vi "GPIB with VISA functions2.vi"() -> ()   [LabVIEW 2015]
doc: "本范例需要在系统中安装NI-488.2和NI-VISA。本范例演示了如何通过对返回数据使用VISA读取、写入和格式函数，与GPIB仪器进行通信。本范例可用于NI Instrument Simulator或其他类似仪器。"
panel:
  in  "波形":enum16{"SIN", "SQU", "RAND"}(ring)
  out "波形图":dbl[](graph)
  out "原始数据":string
  in  "VISA GPIB资源":refnum<visa-resource-name>="GPIB0::2::INSTR"
  # "概述：演示使用VISA函数与GPIB仪器进行通信的方法。\n要求：NI-488.2和NI-VISA驱动程序\n操作步骤：\n1. 请先在Measurement & Automation Explorer正确配置VISA GPIB资源控件中指定的资源。\n2. 运行VI。\n3.如仪器识别了\"SOUR:FUNC\"和\"SENS:DATA?\"命令，则应返回指定的波形数据。"
  # "Windows/Linux用户可使用“仪器驱动程序查找器”（帮助>查找仪器驱动）为仪器查找相应的驱动程序。"
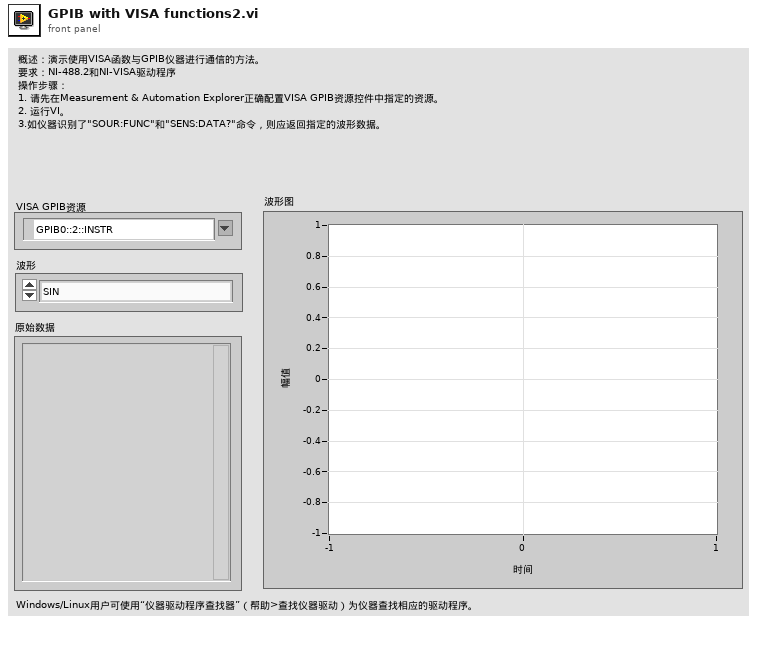
[diagram p1: front panel]
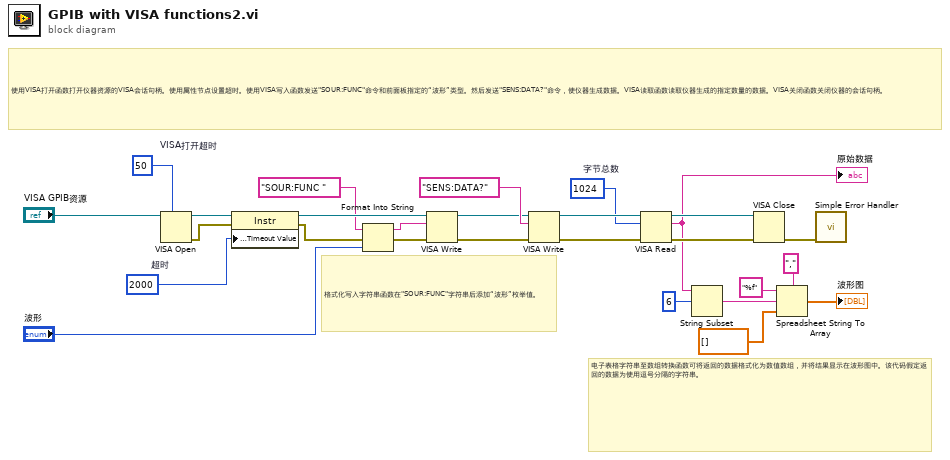
[diagram p0: block diagram]
diagram:
  w17 = u32 1024  # 字节总数
  w22 = u32 2000  # 超时
  w23 = u32 50  # VISA打开超时
  # "电子表格字符串至数组转换函数可将返回的数据格式化为数值数组，并将结果显示在波形图中。该代码假定返回的数据为使用逗号分隔的字符串。"
  # "格式化写入字符串函数在\"SOUR:FUNC\"字符串后添加“波形”枚举值。"
  # "使用VISA打开函数打开仪器资源的VISA会话句柄。使用属性节点设置超时。使用VISA写入函数发送\"SOUR:FUNC\"命令和前面板指定的“波形”类型。然后发送\"SENS:DATA?\"命令，使仪器生成数据。VISA读取函数读取仪器生成的指定数量的数据。VISA关闭函数关闭仪器的会话句柄。"
  n1 = VISA Open(timeout (0)=w23, VISA resource name="VISA GPIB资源") -> (VISA resource name=w21:refnum<visa-resource-name>, error out=w20:errorcluster)  [unwired: 3 in]
  n2 = property class="Instr"(reference=w21, error in=w20, "General Settings:Timeout Value"=w22) -> (reference out=w8:refnum<visa-resource-name>, error out=w4:errorcluster)
  n3 = Format Into String(initial string="SOUR:FUNC " ("string"), error in=w4, "波形") -> (resulting string=w1:string, error out=w3:errorcluster)  [unwired: 1 in]
  n4 = VISA Write(VISA resource name=w8, write buffer=w1, error in (no error)=w3) -> (VISA resource name out=w7:refnum<visa-resource-name>, error out=w6:errorcluster)  [unwired: 1 out]
  n5 = VISA Write(VISA resource name=w7, write buffer="SENS:DATA?" ("Write Buffer"), error in (no error)=w6) -> (VISA resource name out=w27:refnum<visa-resource-name>, error out=w25:errorcluster)  [unwired: 1 out]
  n6 = VISA Read(VISA resource name=w27, byte count=w17, error in (no error)=w25) -> (VISA resource name out=w26:refnum<visa-resource-name>, read buffer=w15:string, error out=w24:errorcluster)  [unwired: 1 out]
  "原始数据" <- w15
  n7 = String Subset(string=w15, offset (0)=6) -> (substring=w13:string)  [unwired: 1 in]
  n8 = VISA Close(VISA resource name=w26, error in (no error)=w24) -> (error out=w16:errorcluster)
  n9 = Spreadsheet String To Array(delimiter (Tab)=",", format string="%f", spreadsheet string=w13, array type (2D Dbl)=dbl[] []) -> (array=→"波形图":dbl[])
  n10 = call <vilib>:"Simple Error Handler.vi"("error in (no error)"=w16) -> ()  [unwired: 4 in, 5 out]
